vi "LaunchCOUI.vi"() -> ()   [LabVIEW 2014, in "zsLaunch.lvlib" / "Launcher.lvclass"]
uses:
  Launcher.lvclass
  <vilib>/ActorFramework/Actor/Actor.lvclass
  CoordinatorUI_lib/State Pattern UI/CoordinatorUI.lvclass
panel:
  out "error out":errorcluster caption="错误输出"
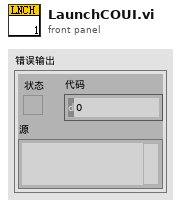
[diagram p1: front panel]
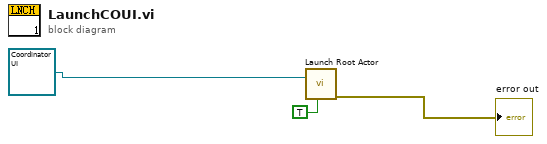
[diagram p0: block diagram]
diagram:
  n1 = call <vilib>:"Launch Root Actor.vi"("Open Actor Core front panel? (F)"=TRUE, "Actor"=refnum<class "CoordinatorUI.lvclass"> refnum ("CoordinatorUI.lvlib:CoordinatorUI.lvclass")) -> ("error out"=→"error out":errorcluster)  [unwired: 8 in, 1 out]
